vi "FlexDDS-NG_DCP_Wait_Event.vi"(4 "Event 2":T1(ring)=enum."NONE", 6 "Event 1":T1(ring)=enum."NONE", 7 "flush?":bool, 8 "AND/OR":enum32{"AND", "OR"}(ring), 9 "waiting time [ms]":dbl, 10 "Channels in":T2(ring)=enum."Both channels", 11 "appended instruction string in":string="dds reset\rdcp spi:STP0=0x3FFF00000CCCCCCD\rdcp spi:CFR1=0x400000\rdcp spi:CFR2=0x80080\rdcp spi:DRL=0x147AE14811EB851F\rdcp spi:DRR=0x400040\rdcp spi:DRSS=0xB0000000B\rdcp update:-d\r") -> (3 "appended instruction string":string="dds reset\rdcp spi:STP0=0x3FFF00000CCCCCCD\rdcp spi:CFR1=0x400000\rdcp spi:CFR2=0x80080\rdcp spi:DRL=0x147AE14811EB851F\rdcp spi:DRR=0x400040\rdcp spi:DRSS=0xB0000000B\rdcp update:-d\rdcp wait:125000h:BNC_IN_A_RISING\r")   [LabVIEW 2016]
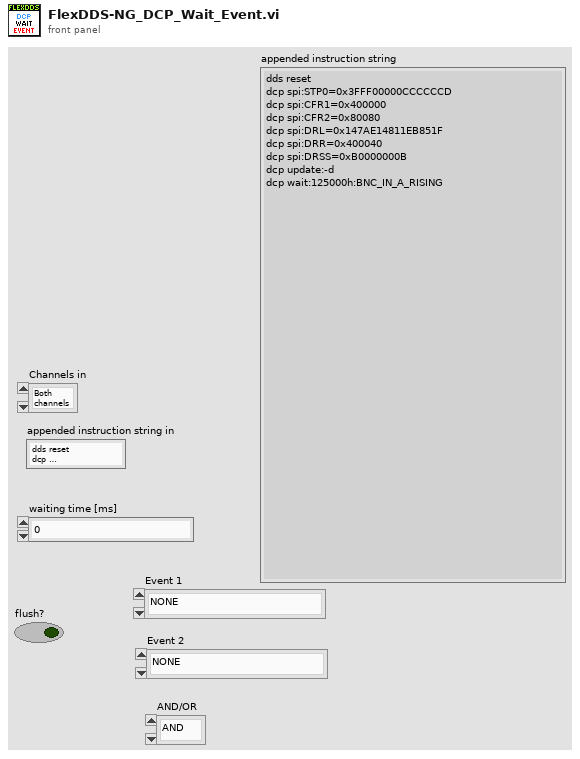
[diagram p1: front panel]
types:
  T1 = enum32{"O_RAMP_SWP_OVR", "RAM_SWP_OVR", "O_DROVER", "DROVER", "O_SPI_FIFO_EV1", "SPI_FIFO_EV1", "O_SPI_FIFO_EV0", "SPI_FIFO_EV0", "O_SPI_FIFO_FLUSHED", "SPI_FIFO_FLUSHED", "BNC_IN_B_LEVEL", "BNC_IN_B_FALLING", "BNC_IN_B_RISING", "BNC_IN_A_LEVEL", "BNC_IN_A_FALLING", "BNC_IN_A_RISING", "ALL_SPI_FIFOS_FLUSHED", "NONE"}
  T2 = enum32{"Channel 0", "Channel 1", "Both channels"}
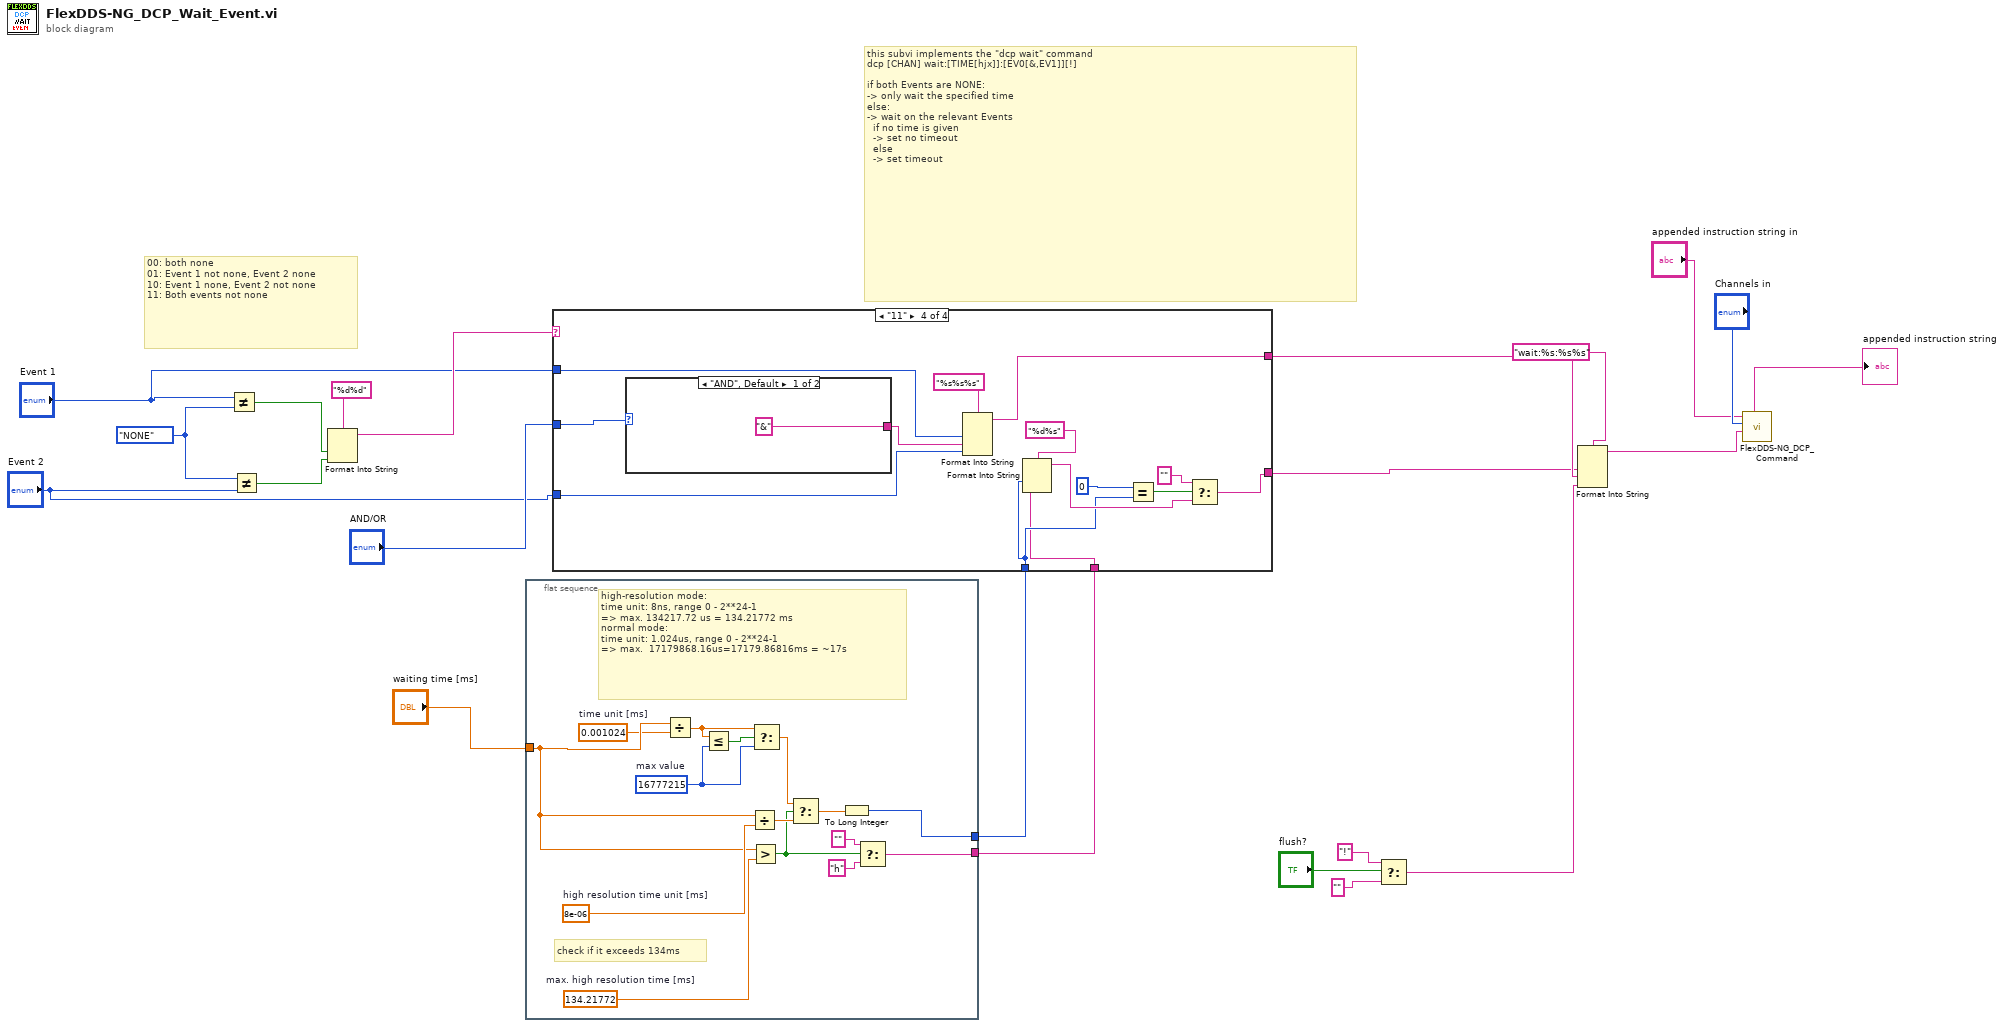
[diagram p0: block diagram]
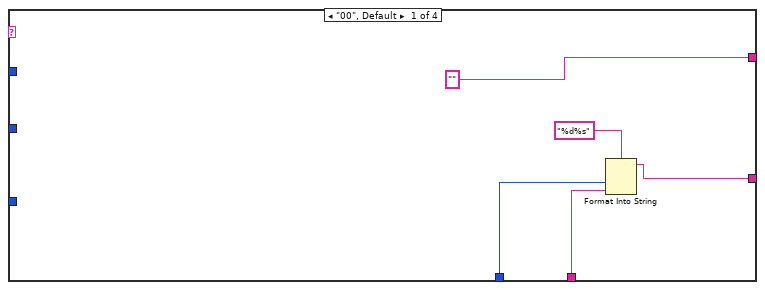
[diagram p2: hidden frame]
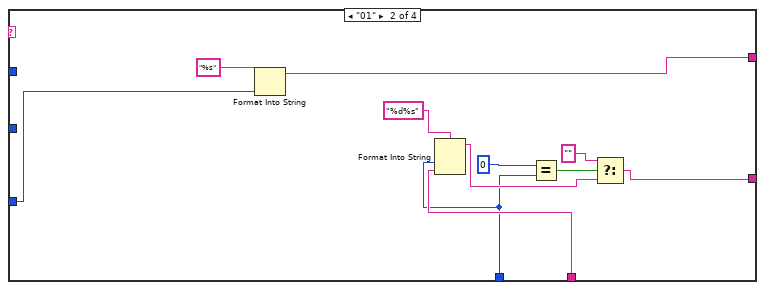
[diagram p3: hidden frame]
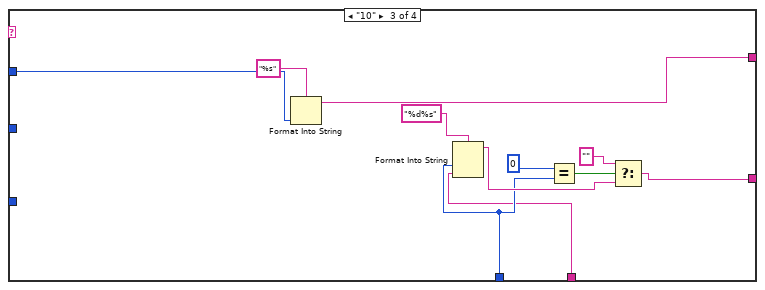
[diagram p4: hidden frame]
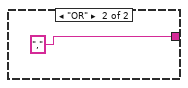
[diagram p5: hidden frame]
diagram:
  w12 = T1."NONE" ("x")
  # "00: both none\n01: Event 1 not none, Event 2 none\n10: Event 1 none, Event 2 not none\n11: Both events not none"
  # "this subvi implements the \"dcp wait\" command\ndcp [CHAN] wait:[TIME[hjx]]:[EV0[&,EV1]][!]\n\nif both Events are NONE:\n-> only wait the specified time\nelse:\n-> wait on the relevant Events\n  if no time is given\n  -> set no timeout\n  else\n  -> set timeout"
  n1 = Not Equal?(x="Event 1", y=w12) -> (x != y?=w11:bool)
  n2 = Not Equal?(x=w12, y="Event 2") -> (x != y?=w10:bool)
  n3 = Format Into String(format string="%d%d", w11, w10) -> (resulting string=w8:string)  [unwired: 2 in, 1 out]
  n4 = flat-sequence {
    tunnel: "waiting time [ms]" -> [w31]
    tunnel: [w23] -> w1
    tunnel: [w24] -> w3
    frame #0 {
      w35 = 16777215  # max value
      w30 = 0.001024  # time unit [ms]
      w32 = 8e-06  # high resolution time unit [ms]
      w28 = 134.21772  # max. high resolution time [ms]
      # "check if it exceeds 134ms"
      # "high-resolution mode:\ntime unit: 8ns, range 0 - 2**24-1\n=> max. 134217.72 us = 134.21772 ms\nnormal mode:\ntime unit: 1.024us, range 0 - 2**24-1\n=> max.  17179868.16us=17179.86816ms = ~17s"
      n5 = Divide(x=w31, y=w30) -> (x/y=w37:dbl)
      n6 = Less Or Equal?(x=w37, y=w35) -> (x <= y?=w34:bool)
      n7 = Divide(x=w31, y=w32) -> (x/y=w33:dbl)
      n8 = Greater?(x=w31, y=w28) -> (0:w27:bool)
      n9 = Select(t=w37, s=w34, f=w35) -> (s? t:f=w36:dbl)
      n10 = Select(t=w36, s=w27, f=w33) -> (s? t:f=w29:dbl)
      n11 = To Long Integer(number=w29) -> (32bit integer=w23:i32)
      n12 = Select(t="", s=w27, f="h") -> (s? t:f=w24:string)
    }
  }
  n13 = case shown="\"11\"" w8 {
    tunnel: "AND/OR" -> [_ _ _ w78]
    tunnel: ["" w51 w63 w74] -> w7
    tunnel: "Event 1" -> [_ _ w64 w77]
    tunnel: "Event 2" -> [_ w52 _ w75]
    tunnel: w1 -> [w40 w43 w55 w67]
    tunnel: w3 -> [w39 w44 w54 w66]
    tunnel: [w41 w47 w56 w68] -> w2
    frame "00", Default {
      n14 = Format Into String(format string="%d%s", w40, w39) -> (resulting string=w41:string)  [unwired: 2 in, 1 out]
    }
    frame "01" {
      n15 = Format Into String(format string="%s", w52) -> (resulting string=w51:string)  [unwired: 2 in, 1 out]
      n16 = Format Into String(format string="%d%s", w43, w44) -> (resulting string=w45:string)  [unwired: 2 in, 1 out]
      n17 = Equal?(x=0, y=w43) -> (x = y?=w49:bool)
      n18 = Select(t="", s=w49, f=w45) -> (s? t:f=w47:string)
    }
    frame "10" {
      n19 = Format Into String(format string="%s", w64) -> (resulting string=w63:string)  [unwired: 2 in, 1 out]
      n20 = Format Into String(format string="%d%s", w55, w54) -> (resulting string=w61:string)  [unwired: 2 in, 1 out]
      n21 = Equal?(x=0, y=w55) -> (x = y?=w58:bool)
      n22 = Select(t="", s=w58, f=w61) -> (s? t:f=w56:string)
    }
    frame "11" {
      n23 = case shown="\"AND\", Default" w78 {
        tunnel: ["&" ","] -> w76
        frame "AND", Default {
        }
        frame "OR" {
        }
      }
      n24 = Format Into String(format string="%s%s%s", w77, w76, w75) -> (resulting string=w74:string)  [unwired: 2 in, 1 out]
      n25 = Format Into String(format string="%d%s", w67, w66) -> (resulting string=w69:string)  [unwired: 2 in, 1 out]
      n26 = Equal?(x=0, y=w67) -> (x = y?=w72:bool)
      n27 = Select(t="", s=w72, f=w69) -> (s? t:f=w68:string)
    }
  }
  n28 = Select(t="!", s="flush?", f="") -> (s? t:f=w6:string)
  n29 = Format Into String(format string="wait:%s:%s%s", w2, w7, w6) -> (resulting string=w13:string)  [unwired: 2 in, 1 out]
  n30 = call "FlexDDS-NG_DCP_Command.vi"("command string"=w13, "Channels"="Channels in", "initial instruction string"="appended instruction string in") -> ("appended instruction string"=→"appended instruction string":string)  [unwired: 8 in]
